vi "Periodic Linear Combination of 1-Exp Distributed Random Variable.vi"(5 "a 1 (in [0, 1])":dbl min=0.0 max=1.0, 6 "seed (-1)":i32=-1, 7 "tau 2":dbl min=0.0, 8 "Error In":errorcluster, 9 "T":dbl min=0.0, 10 "tau 1":dbl min=0.0, 11 "# Elements":i32) -> (0 "Error Out":errorcluster, 3 "t Array":dbl[](array[numeric]))   [LabVIEW 2021, in "Math.lvlib"]
uses:
  Math.lvlib
  AlliGator/Fit Method Benchmark/AlliGator 2-Exp Parameters.ctl
  <vilib>/Utility/error.llb/Error Cluster From Error Code.vi
  <vilib>/gmath/statdist.llb/Uniform Random.vi
  <vilib>/ErrorRing/Error Ring.xnode
  <vilib>/gmath/NI_Gmath.lvlib
  Error/Error.lvlib
  Comparison/Comparison.lvlib
  AlliGator/Fit Method Benchmark/AlliGator Fit Method Benchmark.lvlib
panel:
  # "f(t) = A_1 exp(-t/tau_1) + A_2 exp(-t/tau_2)\nf_1 = A_1/(A_1 + A_2)"
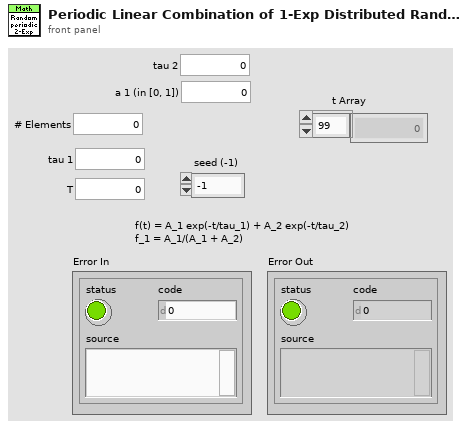
[diagram p1: front panel]
types:
  T1 = typedef "AlliGator Fit Method Benchmark.lvlib/AlliGator 2-Exp Parameters.ctl" = cluster{"tau 1":dbl, "tau 2":dbl, "T":dbl}
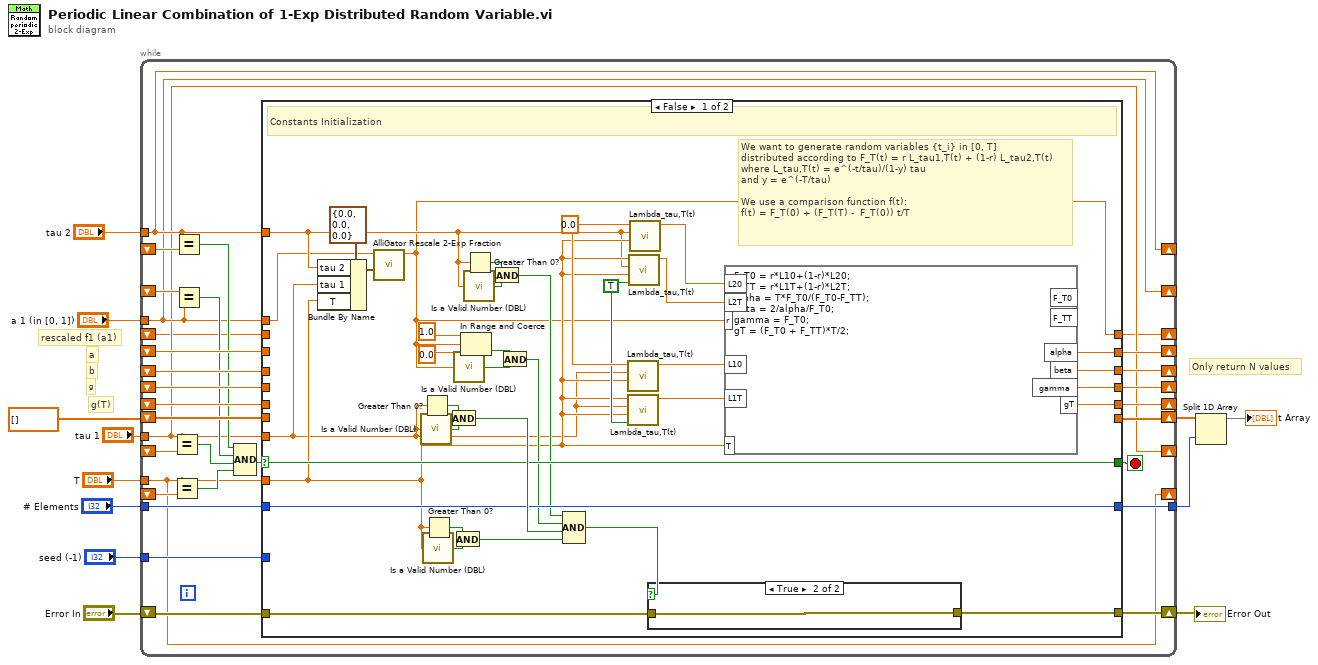
[diagram p0: block diagram]
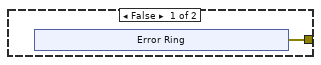
[diagram p2: hidden frame]
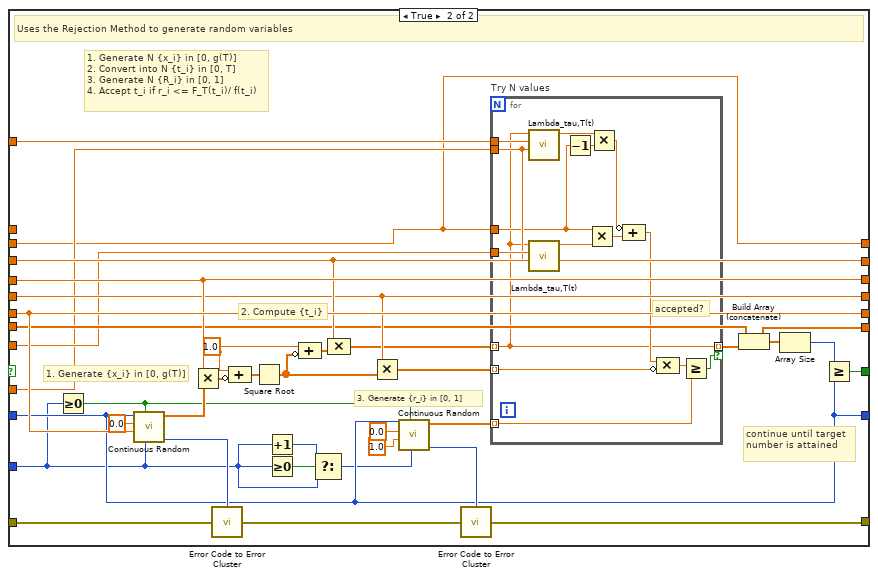
[diagram p3: hidden frame]
diagram:
  # "rescaled f1 (a1)"
  # "Only return N values"
  # "a"
  # "g"
  # "b"
  # "g(T)"
  n1 = while {
    tunnel: "tau 1" -> [w18]
    tunnel: "T" -> [w15]
    shift-right: [w42] -> _
    shift-left: _ -> [w41]
    tunnel: "# Elements" -> [w40]
    shift-right: [w39] -> _
    shift-left: _ -> [w37]
    shift-right: [w38] -> _
    shift-left: _ -> [w36]
    shift-right: [w33] -> w7
    shift-left: "Error In" -> [w34]
    shift-right: [w32] -> _
    shift-left: _ -> [w31]
    shift-right: [w28] -> w6
    shift-left: dbl[] [] -> [w29]
    tunnel: [w27] -> w5
    tunnel: "a 1 (in [0, 1])" -> [w21]
    tunnel: "tau 2" -> [w25]
    shift-right: [w25] -> _
    shift-left: _ -> [w26]
    shift-right: [w21] -> _
    shift-left: _ -> [w22]
    shift-right: [w18] -> _
    shift-left: _ -> [w20]
    shift-right: [w15] -> _
    shift-left: _ -> [w17]
    shift-right: [w14] -> _
    shift-left: _ -> [w13]
    tunnel: "seed (-1)" -> [w35]
    stop <- w30 stop-if-true
    n2 = Equal?(x=w18, y=w20) -> (x = y?=w19:bool)
    n3 = Equal?(x=w15, y=w17) -> (x = y?=w16:bool)
    n4 = Equal?(x=w25, y=w26) -> (x = y?=w24:bool)
    n5 = Equal?(x=w22, y=w21) -> (x = y?=w23:bool)
    n6 = Compound Arithmetic op=AND(w24, w23, w19, w16) -> (w43:bool)
    n7 = case shown="False" w43 {
      selector: w43 -> [w66 _]
      tunnel: w18 -> [w46 w94]
      tunnel: w15 -> [w48 w92]
      tunnel: [w79 w120] -> w42
      tunnel: w41 -> [_ w120]
      tunnel: w40 -> [w65 w98]
      tunnel: [w78 w118] -> w39
      tunnel: [w77 w110] -> w38
      tunnel: w37 -> [_ w118]
      tunnel: w36 -> [_ w110]
      tunnel: w35 -> [_ w87]
      tunnel: w34 -> [w69 w97]
      tunnel: [w68 w100] -> w33
      tunnel: [w67 w111] -> w32
      tunnel: w31 -> [_ w111]
      tunnel: [w66 w106] -> w30
      tunnel: w29 -> [_ w108]
      tunnel: [_ w105] -> w28
      tunnel: [w65 w98] -> w27
      tunnel: w25 -> [w47 w93]
      tunnel: w21 -> [w45 _]
      tunnel: [w44 w91] -> w14
      tunnel: w13 -> [_ w91]
      frame False {
        w51 = TRUE ("T-?")
        w59 = 0.0 ("t")
        # "We want to generate random variables {t_i} in [0, T]\ndistributed according to F_T(t) = r L_tau1,T(t) + (1-r) L_tau2,T(t)\nwhere L_tau,T(t) = e^(-t/tau)/(1-y) tau\nand y = e^(-T/tau)\n\nWe use a comparison function f(t):\nf(t) = F_T(0) + (F_T(T) -  F_T(0)) t/T"
        # "Constants Initialization"
        n8 = Bundle By Name(cluster=T1 {"tau 1"=0.0, "tau 2"=0.0, "T"=0.0} ("2-Exp Parameters"), "tau 2"=w47, "tau 1"=w46, "T"=w48) -> (w50:T1)
        n9 = call "AlliGator Rescale 2-Exp Fraction.vi"("2-Exp Parameters"=w50, "a 1 in"=w45) -> ("r 1 out"=w44:dbl)  [unwired: 9 in]
        n10 = call "Is a Valid Number (DBL).vi"("Number"=w46) -> ("Valid Number?"=w75:bool)  [unwired: 8 in]
        n11 = Greater Than 0?(x=w46) -> (x > 0?=w76:bool)
        n12 = call "Is a Valid Number (DBL).vi"("Number"=w48) -> ("Valid Number?"=w73:bool)  [unwired: 8 in]
        n13 = Greater Than 0?(x=w48) -> (x > 0?=w74:bool)
        n14 = And(x=w76, y=w75) -> (x .and. y?=w71:bool)
        n15 = And(x=w74, y=w73) -> (x .and. y?=w72:bool)
        n16 = call "Is a Valid Number (DBL).vi"("Number"=w44) -> ("Valid Number?"=w64:bool)  [unwired: 8 in]
        n17 = In Range and Coerce(upper limit=1.0, x=w44, lower limit=0.0) -> (In Range?=w52:bool)  [unwired: 1 out]
        n18 = call "Is a Valid Number (DBL).vi"("Number"=w47) -> ("Valid Number?"=w62:bool)  [unwired: 8 in]
        n19 = Greater Than 0?(x=w47) -> (x > 0?=w61:bool)
        n20 = And(x=w61, y=w62) -> (x .and. y?=w60:bool)
        n21 = And(x=w52, y=w64) -> (x .and. y?=w63:bool)
        n22 = Compound Arithmetic op=AND(w60, w63, w71, w72) -> (w70:bool)
        n23 = call "Lambda_tau,T(t).vi"("T"=w48, "tau"=w46, "t"=w59) -> ("Lambda_[tau,T](t)"=w56:dbl)  [unwired: 8 in]
        n24 = call "Lambda_tau,T(t).vi"("T-?"=w51, "T"=w48, "tau"=w46, "t"=w48) -> ("Lambda_[tau,T](t)"=w55:dbl)  [unwired: 7 in]
        n25 = call "Lambda_tau,T(t).vi"("T-?"=w51, "T"=w48, "tau"=w47, "t"=w48) -> ("Lambda_[tau,T](t)"=w57:dbl)  [unwired: 7 in]
        n26 = call "Lambda_tau,T(t).vi"("T"=w48, "tau"=w47, "t"=w59) -> ("Lambda_[tau,T](t)"=w58:dbl)  [unwired: 8 in]
        n27 = case shown="True" w70 {
          tunnel: w69 -> [_ w85]
          tunnel: [w80 w85] -> w68
          frame False {
            n28 = xnode "Error Ring"() -> ("error out"=w80:errorcluster)
          }
          frame True {
          }
        }
        n29 = formula code="F_T0 = r*L10+(1-r)*L20;\nF_TT = r*L1T+(1-r)*L2T;\nalpha = T*F_T0/(F_T0-F_TT);\nbeta = 2/alpha/F_T0;\ngamma = F_T0;\ngT = (F_T0 + F_TT)*T/2;"("T"=w48, "L10"=w56, "L1T"=w55, "L20"=w58, "L2T"=w57, "r"=w44) -> ("gT"=w79:dbl, "beta"=w78:dbl, "gamma"=w77:dbl, "alpha"=w67:dbl)  [unwired: 2 out]
      }
      frame True {
        w113 = 1.0 ("xmin")
        # "3. Generate {r_i} in [0, 1]"
        # "2. Compute {t_i}"
        # "1. Generate {x_i} in [0, g(T)]"
        # "1. Generate N {x_i} in [0, g(T)]\n2. Convert into N {t_i} in [0, T]\n3. Generate N {R_i} in [0, 1]\n4. Accept t_i if r_i <= F_T(t_i)/ f(t_i)"
        # "continue until target number is attained"
        # "Uses the Rejection Method to generate random variables"
        n30 = Greater Or Equal To 0?(x=w87) -> (x >= 0?=w86:bool)
        n31 = call-poly <vilib>:"Continuous Random.vi"("seed"=w87, "reset"=w86, "xmax"=w120, "xmin"=0.0, "samples"=w98) -> ("error"=w115:i32, "uniform random data"=w119:dbl[])  [unwired: 5 in]
        n32 = Multiply(x=w118, y=w119) -> (x*y=w117:dbl[])
        n33 = call "Error Code to Error Cluster.vi"("Error Code"=w115, "Error In"=w97) -> ("Error Out"=w96:errorcluster)  [unwired: 13 in]
        n34 = Compound Arithmetic op=ADD(w113, invert w117) -> (w116:dbl[])
        n35 = Square Root(x=w116) -> (sqrt(x)=w114:dbl[])
        n36 = Increment(x=w87) -> (x+1=w88:i32)
        n37 = Greater Or Equal To 0?(x=w87) -> (x >= 0?=w90:bool)
        n38 = Compound Arithmetic op=ADD(w113, invert w114) -> (w112:dbl[])
        n39 = Select(t=w88, s=w90, f=w87) -> (s? t:f=w89:i32)
        n40 = Compound Arithmetic op=MULTIPLY(w111, w112) -> (w104:dbl[])
        n41 = Multiply(x=w110, y=w114) -> (x*y=w95:dbl[])
        n42 = call-poly <vilib>:"Continuous Random.vi"("seed"=w89, "reset"=w86, "xmax"=1.0, "xmin"=0.0 ("xmax"), "samples"=w98) -> ("error"=w101:i32, "uniform random data"=w102:dbl[])  [unwired: 5 in]
        n43 = call "Error Code to Error Cluster.vi"("Error Code"=w101, "Error In"=w96) -> ("Error Out"=w100:errorcluster)  [unwired: 13 in]
        n44 = for "Try N values" {
          tunnel: [w122] -> w109 mode=indexing if=w136
          tunnel: w104 -> [w122] mode=indexing
          tunnel: w102 -> [w131] mode=indexing
          tunnel: w95 -> [w135] mode=indexing
          tunnel: w94 -> [w133]
          tunnel: w93 -> [w132]
          tunnel: w92 -> [w130]
          tunnel: w91 -> [w127]
          # "accepted?"
          n45 = call "Lambda_tau,T(t).vi"("T"=w130, "tau"=w132, "t"=w122) -> ("Lambda_[tau,T](t)"=w128:dbl)  [unwired: 8 in]
          n46 = call "Lambda_tau,T(t).vi"("T"=w130, "tau"=w133, "t"=w122) -> ("Lambda_[tau,T](t)"=w129:dbl)  [unwired: 8 in]
          n47 = Decrement(x=w127) -> (x-1=w126:dbl)
          n48 = Multiply(x=w127, y=w129) -> (x*y=w125:dbl)
          n49 = Multiply(x=w128, y=w126) -> (x*y=w124:dbl)
          n50 = Compound Arithmetic op=ADD(invert w124, w125) -> (w123:dbl)
          n51 = Compound Arithmetic op=MULTIPLY(w123, invert w135) -> (w134:dbl)
          n52 = Greater Or Equal?(x=w134, y=w131) -> (x >= y?=w136:bool)
        }
        n53 = Build Array (concatenate)(w108, w109) -> (w105:dbl[])
        n54 = Array Size(array=w105) -> (size(s)=w107:i32)
        n55 = Greater Or Equal?(x=w107, y=w98) -> (x >= y?=w106:bool)
      }
    }
  }
  "Error Out" <- w7
  n56 = Split 1D Array(array=w6, index=w5) -> (first subarray=→"t Array":dbl[])  [unwired: 1 out]
